vi "Check is Work VI.vi"(11 "Item Refnum":refnum<vi>) -> (3 "Work VI?":bool)   [LabVIEW 2020, in "FlexWorker_Provider.lvlib"]
uses:
  FlexWorker_Provider.lvlib
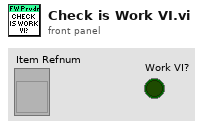
[diagram p1: front panel]
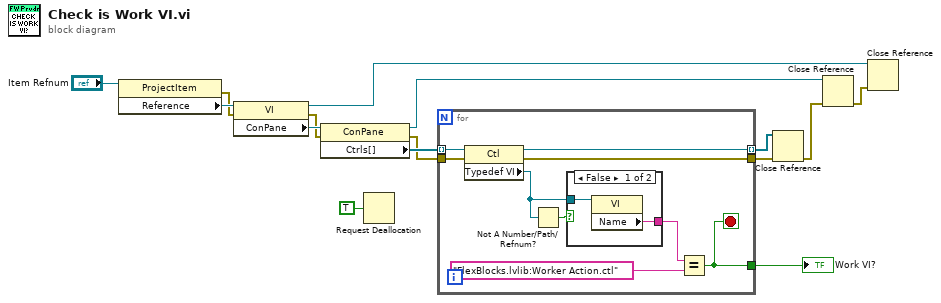
[diagram p0: block diagram]
diagram:
  n1 = property class="ProjectItem"(reference="Item Refnum") -> (error out=w10:errorcluster, "Reference"=w14:refnum<vi>)  [unwired: 1 in, 1 out]
  n2 = property class="VI"(reference=w14, error in=w10) -> (reference out=w1:refnum<vi>, error out=w9:errorcluster, "ConPane"=w13:refnum<vi>)
  n3 = property class="ConPane"(reference=w13, error in=w9) -> (reference out=w3:refnum<vi>, error out=w8:errorcluster, "Ctrls[]"=w11:refnum<vi>[])
  n4 = Request Deallocation(TRUE ("flag")) -> ()
  n5 = for {
    tunnel: w11 -> [w24] mode=indexing
    tunnel: [w21] -> w7
    tunnel: [w20] -> w5 mode=indexing
    tunnel: w8 -> [w19]
    tunnel: [w16] -> w6
    stop <- w21 stop-if-true
    n6 = property class="Ctl"(reference=w24, error in=w19) -> (reference out=w20:refnum<vi>, error out=w16:errorcluster, "Typedef VI"=w18:refnum<vi>)
    n7 = Not A Number/Path/Refnum?(number/path/refnum=w18) -> (NaN/Path/Refnum?=w17:bool)
    n8 = case shown="False" w17 {
      tunnel: [w26 _] -> w23
      tunnel: w18 -> [w25 _]
      frame False {
        n9 = property class="VI"(reference=w25) -> ("Name"=w26:string)  [unwired: 1 in, 2 out]
      }
      frame True {
      }
    }
    n10 = Equal?(x=w23, y="FlexBlocks.lvlib:Worker Action.ctl") -> (x = y?=w21:bool)
  }
  "Work VI?" <- w7
  n11 = Close Reference(reference=w5, error in (no error)=w6) -> (error out=w4:errorcluster)
  n12 = Close Reference(reference=w3, error in (no error)=w4) -> (error out=w2:errorcluster)
  n13 = Close Reference(reference=w1, error in (no error)=w2) -> ()  [unwired: 1 out]
